vi "Periodic Tasks.vi"(8 "error in":errorcluster) -> ()   [LabVIEW 2012]
doc: "This VI runs in parallel to other tasks. It can contain as many user-defined periodic loops as you need. These can carry out PID or other sorts of timed response."
uses:
  RefnameEnum.ctl
  QueueEnum.ctl
  TankDriveInstruction.ctl
  <vilib>/Rock Robotics/SystemInterfaces/Utilities/FPGA_UtilitiesLED Source.ctl
  <vilib>/Rock Robotics/SystemInterfaces/Utilities/FPGA_UtilitiesLED State.ctl
  <vilib>/Rock Robotics/WPI/Compressor/WPI_CompressorGetSetRefNum.vi
  Robot Global Data.vi
  <vilib>/Rock Robotics/WPI/RobotDrive/WPI_RobotDriveGetSetRefNum.vi
panel:
  out "Compressor Loop Running":bool
  out "Compressor Running":bool
  out "Compressor Enabled":bool
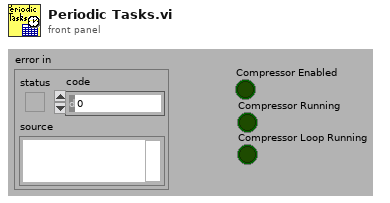
[diagram p1: front panel]
types:
  T1 = typedef "RefnameEnum.ctl" = enum16{"FireLauncher", "Climber", "Shield", "TankDrive", "DriveEncoderL", "DriveEncoderR", "LauncherMotorRPM", "LauncherEncoderAnalog", "LauncherEncoderRPM", "ShooterLS", "DriveAlignLSLeft", "DriveAlignLSRight", "ClimbingLS", "LauncherEncoderAngle", "LauncherMotorAngle", "Gamepad1", "Gamepad2", "Compressor", "ClimbWeightSol3", "ClimbWeightSol4"}
  T2 = typedef "QueueEnum.ctl" = enum16{"cTankDrive", "cClimb", "cLauncherAngle", "cLauncherWheel", "cFirePneumatic"}
  T3 = typedef "FPGA_UtilitiesLED State.ctl" = enum16{"Off", "On", "Toggle"}
  T4 = typedef "FPGA_UtilitiesLED Source.ctl" = enum16{"User LED", "FPGA LED"}
  T5 = typedef "WPI_CompressorDevRef.ctl" = cluster{"DevStatus":errorcluster, "DigitalInputDevRef":T6, "RelayDevRef":T9}
  T6 = typedef "WPI_DigitalInputDevRef.ctl" = cluster{"DevStatus":errorcluster, "DIO Channel":T7, "Digital Module":T8}
  T7 = typedef "FPGA_DIOChannel.ctl" = enum8{"DIO 1", "DIO 2", "DIO 3", "DIO 4", "DIO 5", "DIO 6", "DIO 7", "DIO 8", "DIO 9", "DIO 10", "DIO 11", "DIO 12", "DIO 13", "DIO 14", "Invalid"}
  T8 = typedef "FPGA_TypedefDigitalModule.ctl" = enum16{"Digital Module 1", "Digital Module 2"}
  T9 = typedef "WPI_RelayDevRef.ctl" = cluster{"DevStatus":errorcluster, "Relay Channel":T10, "Digital Module":T8, "Relay Direction":T11}
  T10 = typedef "FPGA_DIORelayChannel.ctl" = enum8{"Relay 1", "Relay 2", "Relay 3", "Relay 4", "Relay 5", "Relay 6", "Relay 7", "Relay 8", "Invalid"}
  T11 = typedef "WPI_RelayDirection.ctl" = enum16{"Both directions", "Forward only", "Reverse only"}
  T12 = typedef "WPI_RobotDriveDevRef.ctl" = cluster{"DevStatus":errorcluster, "Motors[]":T13[], "Square Inputs":bool, "Max Output":dbl, "Isochronous":bool}
  T13 = typedef "WPI_MotorControlDeviceRef.ctl" = cluster{"DeviceStatus":errorcluster, "Type":enum16{"PWM", "CAN"}, "PWM":cluster{"Digital Module":T8, "PWM Channel":T14, "DeadBand":T15}, "CAN":cluster{"Device Number":u8, "Control Mode":T16, "Semaphore":T17, "Max Vout":dbl}, "Invert":bool, "TransformRef":T18, "InvTransformRef":T18}
  T14 = typedef "FPGA_DIOPWMChannel.ctl" = enum8{"PWM 1", "PWM 2", "PWM 3", "PWM 4", "PWM 5", "PWM 6", "PWM 7", "PWM 8", "PWM 9", "PWM 10", "Invalid"}
  T15 = typedef "WPI_PWMDeadband.ctl" = cluster{"Name":string, "maxPositivePwm":i32, "minPositivePwm":i32, "centerPwm":i32, "maxNegativePwm":i32, "minNegativePwm":i32, "angularRange":u16}
  T16 = typedef "WPI_CANJaguar_ControlMode.ctl" = enum8{"Percent VBus", "Current", "Speed", "Position", "Voltage"}
  T17 = typedef "Semaphore RefNum" = refnum<k1>
  T18 = typedef "WPI_PWMTransform_ConPane.ctl" = refnum<vi>
  T19 = typedef "TankDriveInstruction.ctl" = cluster{"LeftMotorValue":dbl, "RightMotorValue":dbl, "HalfSpeed":bool}
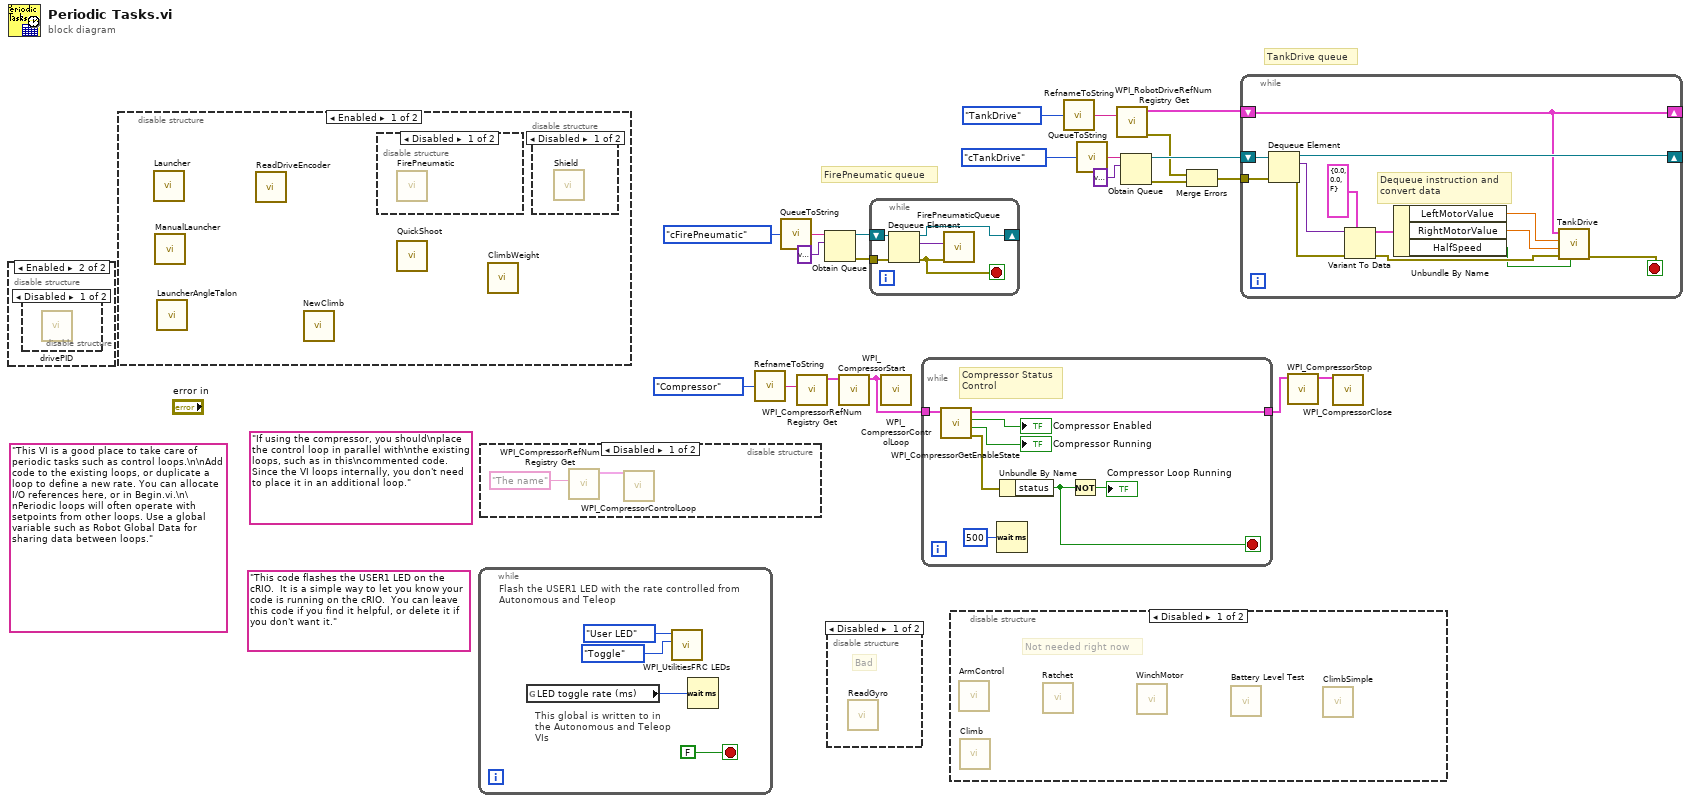
[diagram p0: block diagram]
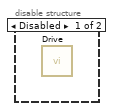
[diagram p2: hidden frame]
diagram:
  (unwired) "If using the compressor, you should\nplace the control loop in parallel with\nthe existing loops, such as in this\ncommented code. Since the VI loops internally, you don't need to place it in an additional loop."
  (unwired) "This code flashes the USER1 LED on the cRIO.  It is a simple way to let you know your code is running on the cRIO.  You can leave this code if you find it helpful, or delete it if you don't want it."
  (unwired) "This VI is a good place to take care of periodic tasks such as control loops.\n\nAdd code to the existing loops, or duplicate a loop to define a new rate. You can allocate I/O references here, or in Begin.vi.\n\nPeriodic loops will often operate with setpoints from other loops. Use a global variable such as Robot Global Data for sharing data between loops."
  # "TankDrive queue"
  # "FirePneumatic queue"
  n1 = disable-structure shown="Enabled" {
    frame Disabled {
      n2 = call "Drive.vi"() -> ()  [unwired: 12 in]
    }
    frame Enabled {
      n3 = disable-structure shown="Disabled" {
        frame Disabled {
          n4 = call "drivePID.vi"() -> ()  [unwired: 12 in]
        }
        frame Enabled {
        }
      }
    }
  }
  n5 = disable-structure shown="Enabled" {
    frame Enabled {
      n6 = call "Launcher.vi"() -> ()  [unwired: 12 in]
      n7 = call "ManualLauncher.vi"() -> ()  [unwired: 12 in]
      n8 = call "LauncherAngleTalon.vi"() -> ()  [unwired: 12 in]
      n9 = call "ReadDriveEncoder.vi"() -> ()  [unwired: 12 in]
      n10 = call "NewClimb.vi"() -> ()  [unwired: 12 in]
      n11 = disable-structure shown="Disabled" {
        frame Disabled {
          n12 = call "FirePneumatic.vi"() -> ()  [unwired: 12 in]
        }
        frame Enabled {
        }
      }
      n13 = call "QuickShoot.vi"() -> ()  [unwired: 12 in]
      n14 = call "ClimbWeight.vi"() -> ()  [unwired: 12 in]
      n15 = disable-structure shown="Disabled" {
        frame Disabled {
          n16 = call "Shield.vi"() -> ()  [unwired: 12 in]
        }
        frame Enabled {
        }
      }
    }
    frame Disabled {
    }
  }
  n17 = while {
    stop <- FALSE stop-if-true
    # "This global is written to in the Autonomous and Teleop VIs"
    # "Flash the USER1 LED with the rate controlled from Autonomous and Teleop"
    n18 = global read "Robot Global Data.vi" "LED toggle rate (ms)"() -> (w22:u32)
    n19 = call <vilib>:"WPI_UtilitiesFRC LEDs.vi"("State"=FPGA_UtilitiesLED_State."Toggle", "LED Type"=FPGA_UtilitiesLED_Source."User LED") -> ()  [unwired: 1 in, 9 out]
    n20 = Wait (ms)(milliseconds to wait=w22) -> ()  [unwired: 1 out]
  }
  n21 = disable-structure shown="Disabled" {
    frame Disabled {
      n22 = call <vilib>:"WPI_CompressorRefNum Registry Get.vi"("refnum name"="The name") -> ("CompressorDevRef"=w27:T5)  [unwired: 9 in, 1 out]
      n23 = call <vilib>:"WPI_CompressorControlLoop.vi"("CompressorDevRef"=w27) -> ()  [unwired: 11 in]
    }
    frame Enabled {
    }
  }
  n24 = call "RefnameToString.vi"("Enum"=RefnameEnum."Compressor") -> ("Refname"=w16:string)
  n25 = call "QueueToString.vi"("QueueEnum"=QueueEnum."cFirePneumatic" ("Queue")) -> ("String"=w11:string)
  n26 = call <vilib>:"WPI_CompressorRefNum Registry Get.vi"("refnum name"=w16) -> ("CompressorDevRef"=w21:T5)  [unwired: 9 in, 1 out]
  n27 = Obtain Queue(name (unnamed)=w11, element data type=variant) -> (queue out=w15:refnum<queue>, error out=w14:errorcluster)  [unwired: 3 in, 1 out]
  n28 = disable-structure shown="Disabled" {
    frame Disabled {
      # "Bad"
      n29 = call "ReadGyro.vi"() -> ()  [unwired: 12 in]
    }
    frame Enabled {
    }
  }
  n30 = call <vilib>:"WPI_CompressorStart.vi"("CompressorDevRef"=w21) -> ("CompressorDevRef"=w20:T5)  [unwired: 9 in, 1 out]
  n31 = while {
    shift-right: [w31] -> _
    shift-left: w15 -> [w32]
    tunnel: w14 -> [w30]
    stop <- w29 stop-if-true
    n32 = Dequeue Element(queue=w32, error in (no error)=w30) -> (queue out=w31:refnum<queue>, element=w28:variant, error out=w29:errorcluster)  [unwired: 1 in, 1 out]
    n33 = call "FirePneumaticQueue.vi"("error in (no error)"=w29, "Variant"=w28) -> ()  [unwired: 9 in, 1 out]
  }
  n34 = call <vilib>:"WPI_CompressorControlLoop.vi"("CompressorDevRef"=w20) -> ()  [unwired: 11 in]
  n35 = while {
    tunnel: w20 -> [w40]
    tunnel: [w35] -> w19
    stop <- w33 stop-if-true
    # "Compressor Status\nControl"
    n36 = call <vilib>:"WPI_CompressorGetEnableState.vi"("CompressorDevRef"=w40) -> ("error out"=w36:errorcluster, "Compressor Running"=→"Compressor Running":bool, "Enabled"=→"Compressor Enabled":bool, "CompressorDevRef"=w35:T5)  [unwired: 1 in, 6 out]
    n37 = Wait (ms)(milliseconds to wait=u32 500) -> ()  [unwired: 1 out]
    n38 = Unbundle By Name(w36) -> ("status"=w33:bool)
    n39 = Not(x=w33) -> (.not. x?=→"Compressor Loop Running":bool)
  }
  n40 = disable-structure shown="Disabled" {
    frame Disabled {
      # "Not needed right now"
      n41 = call "ArmControl.vi"() -> ()  [unwired: 12 in]
      n42 = call "Climb.vi"() -> ()  [unwired: 12 in]
      n43 = call "Ratchet.vi"() -> ()  [unwired: 12 in]
      n44 = call "WinchMotor.vi"() -> ()  [unwired: 12 in]
      n45 = call "Battery Level Test.vi"() -> ()  [unwired: 12 in]
      n46 = call "ClimbSimple.vi"() -> ()  [unwired: 12 in]
    }
    frame Enabled {
    }
  }
  n47 = call "RefnameToString.vi"("Enum"=RefnameEnum."TankDrive") -> ("Refname"=w5:string)
  n48 = call "QueueToString.vi"("QueueEnum"=QueueEnum."cTankDrive" ("Queue")) -> ("String"=w6:string)
  n49 = call <vilib>:"WPI_RobotDriveRefNum Registry Get.vi"("refnum name"=w5) -> ("error out"=w2:errorcluster, "RobotDriveDevRef"=w4:T12)  [unwired: 9 in]
  n50 = Obtain Queue(name (unnamed)=w6, element data type=variant) -> (queue out=w8:refnum<queue>, error out=w3:errorcluster)  [unwired: 3 in, 1 out]
  n51 = Merge Errors(w2, w3) -> (w1:errorcluster)
  n52 = while {
    shift-right: [w52] -> _
    shift-left: w8 -> [w53]
    shift-right: [w42] -> _
    shift-left: w4 -> [w42]
    tunnel: w1 -> [w41]
    stop <- w46 stop-if-true
    # "Dequeue instruction and\nconvert data"
    n53 = Dequeue Element(queue=w53, error in (no error)=w41) -> (queue out=w52:refnum<queue>, element=w51:variant, error out=w47:errorcluster)  [unwired: 1 in, 1 out]
    n54 = Variant To Data(error in=w47, type=T19 {"LeftMotorValue"=0.0, "RightMotorValue"=0.0, "HalfSpeed"=FALSE} ("TankDriveInstruction"), Variant=w51) -> (data=w49:T19, error out=w48:errorcluster)
    n55 = Unbundle By Name(w49) -> ("LeftMotorValue"=w43:dbl, "RightMotorValue"=w44:dbl, "HalfSpeed"=w45:bool)
    n56 = call "TankDrive.vi"("HalfSpeed"=w45, "Error In (no error)"=w48, "Right Motor Value"=w44, "Left Motor Value"=w43, "RobotDriveDevRef"=w42) -> ("Error Out"=w46:errorcluster)  [unwired: 6 in]
  }
  n57 = call <vilib>:"WPI_CompressorStop.vi"("CompressorDevRef"=w19) -> ("CompressorDevRef"=w18:T5)  [unwired: 1 in, 9 out]
  n58 = call <vilib>:"WPI_CompressorClose.vi"("CompressorDevRef"=w18) -> ()  [unwired: 1 in, 10 out]
